vi "PathOhanaOS.vi"() -> (0 "OhanaOS Path":path)   [LabVIEW 2009]
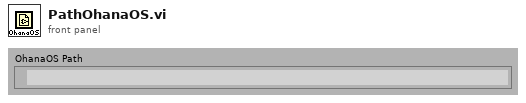
[diagram p1: front panel]
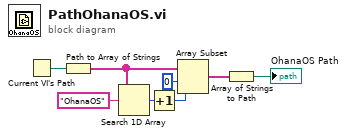
[diagram p0: block diagram]
diagram:
  n1 = Current VI's Path() -> (path=w8:path)
  n2 = Path to Array of Strings(0:w8) -> (2:w6:string[])  [unwired: 1 out]
  n3 = Search 1D Array(1D array=w6, element="OhanaOS" ("élément")) -> (index of element=w5:i32)  [unwired: 1 out]
  n4 = Increment(x=w5) -> (x+1=w2:i32)
  n5 = Array Subset(array=w6, index=0 ("Indice du tableau"), length=w2) -> (w3:string[])
  n6 = Array of Strings to Path(0:w3) -> (2:→"OhanaOS Path":path)  [unwired: 1 out]
